vi "Init State.vi"(5 "Queue in":refnum<queue>, 9 "Test Results in":T1, 11 "error in (no error)":errorcluster) -> (4 ".NET Refnum out":refnum<k24>, 10 "Test Results out":T1, 15 "error out":errorcluster)   [LabVIEW 2016]
doc: "This VI Initializes the GEA2 bus, and sets the reference to the GEA2 Functional Global Variable."
uses:
  C:/Automation/DLLs/PC Dot Net/GeaCommunication.dll
  controls/Test Results.ctl
  C:/Program Files (x86)/National Instruments/LabVIEW 2016/examples/Design Patterns/Queued Message Handler/support/QMH Fundamentals - Message Cluster.ctl
  <vilib>/Utility/error.llb/Error Cluster From Error Code.vi
  <vilib>/ErrorRing/Error Ring.xnode
  Common/LabVIEW GEA2 Toolkit/LabVIEW_GEA2_Toolkit.lvlibp
  Automation/Product Specific/Clothes Care/TL27/Projects/TL27.lvlib
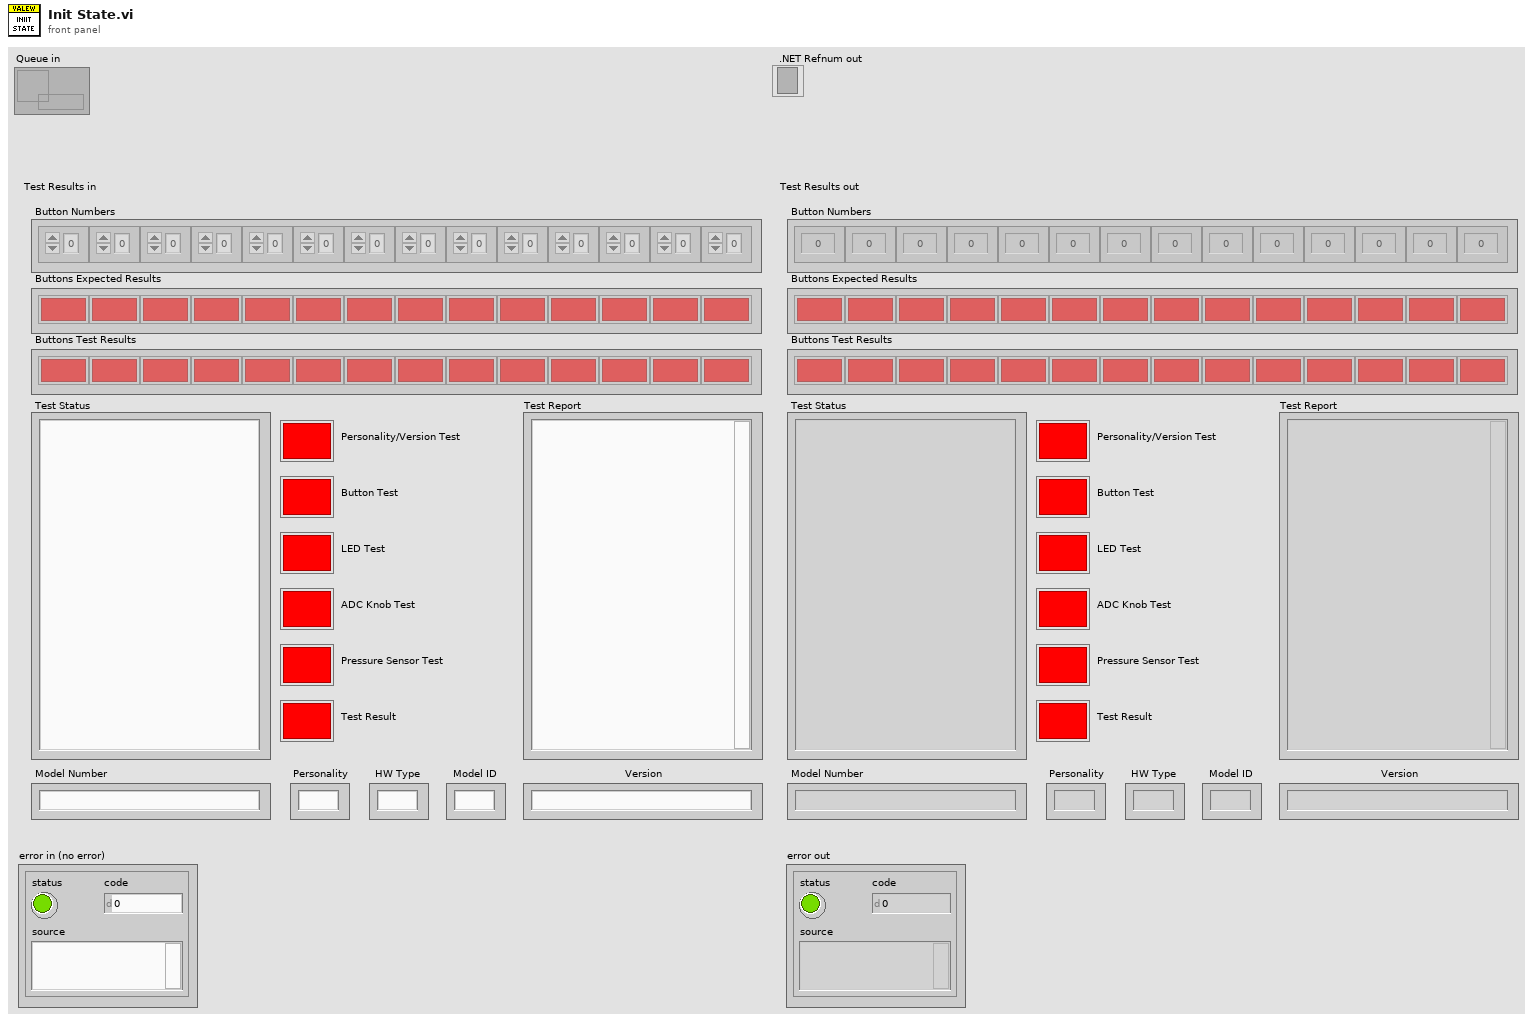
[diagram p1: front panel]
types:
  T1 = typedef "Test Results.ctl" = cluster{"Test Status":string, "Personality/Version Test ":bool, "Test Report":string, "Model Number":string, "Button Numbers":i32[], "Buttons Test Results":bool[], "Buttons Expected Results":bool[], "Model ID":string, "Personality":string, "HW Type":string, "Version":string, "Button Test":bool, "LED Test":bool, "ADC Knob Test":bool, "Pressure Sensor Test":bool, "Test Result":bool}
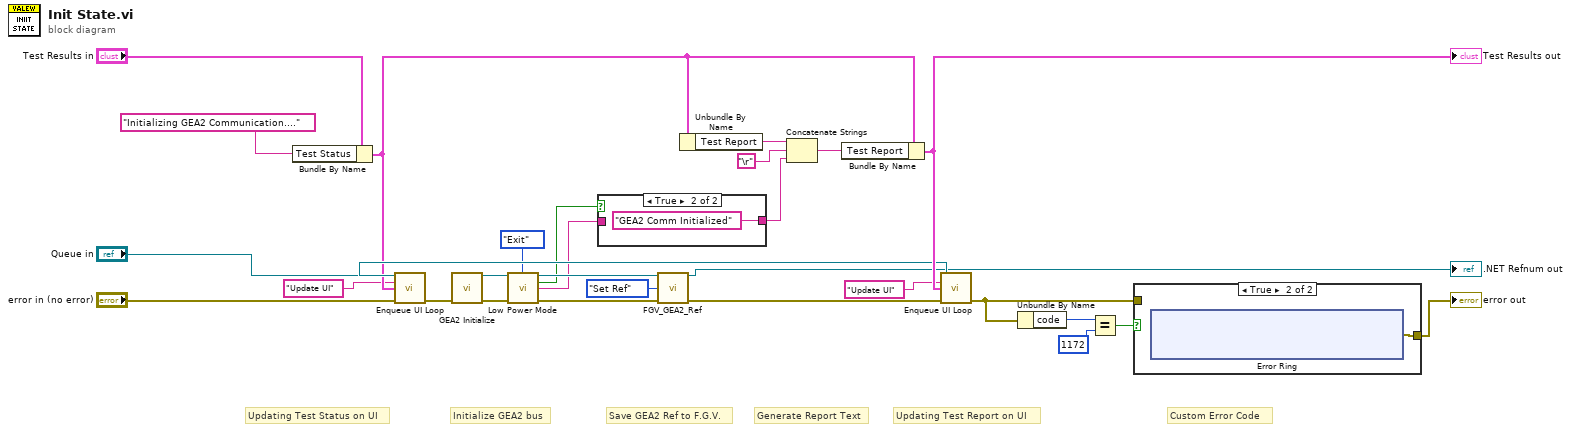
[diagram p0: block diagram]
diagram:
  # "Custom Error Code"
  # "Generate Report Text"
  # "Updating Test Status on UI"
  # "Updating Test Report on UI"
  # "Save GEA2 Ref to F.G.V."
  # "Initialize GEA2 bus"
  n1 = Bundle By Name(cluster="Test Results in", "Test Status"="Initializing GEA2 Communication....") -> (w22:T1)
  n2 = call "Enqueue UI Loop.vi"("UI Que In"="Queue in", "Message"="Update UI", "Test Results"=w22, "error in (no error)"="error in (no error)") -> ("UI Queue Out"=w24:refnum<queue>, "error out"=w20:errorcluster)  [unwired: 10 in]
  n3 = call "GEA2 Initialize.vi"("error in"=w20) -> ("GEA2 Reference Out"=w15:refnum<k24>, "error out"=w16:errorcluster)  [unwired: 12 in, 1 out]
  n4 = call "Low Power Mode.vi"("GEA2 Reference In"=w15, "Action"=enum16{"Enter", "Exit"}."Exit", "Error In"=w16) -> ("GEA2 Reference Out"=w28:refnum<k24>, "Pass/Fail?"=w18:bool, "Report Text"=w19:string, "Error Out"=w23:errorcluster)  [unwired: 9 in]
  n5 = case shown="True" w18 {
    tunnel: [w30 "GEA2 Comm Initialized"] -> w21
    tunnel: w19 -> [w30 _]
    frame False {
    }
    frame True {
    }
  }
  n6 = call "FGV_GEA2_Ref.vi"("GEA2 Reference In"=w28, "Action"=enum16{"Set Ref", "Get Ref"}."Set Ref", "Error In"=w23) -> ("GEA2 Reference Out"=→".NET Refnum out":refnum<k24>, "Error Out"=w27:errorcluster)  [unwired: 11 in]
  n7 = Unbundle By Name(w22) -> ("Test Report"=w9:string)
  n8 = Concatenate Strings(w9, "\r", w21) -> (w7:string)
  n9 = Bundle By Name(cluster=w22, "Test Report"=w7) -> (w26:T1)
  "Test Results out" <- w26
  n10 = call "Enqueue UI Loop.vi"("UI Que In"=w24, "Message"="Update UI", "Test Results"=w26, "error in (no error)"=w27) -> ("error out"=w2:errorcluster)  [unwired: 10 in, 1 out]
  n11 = Unbundle By Name(w2) -> ("code"=w6:i32)
  n12 = Equal?(x=w6, y=1172) -> (x = y?=w4:bool)
  n13 = case shown="True" w4 {
    tunnel: [w32 w33] -> w1
    tunnel: w2 -> [w32 _]
    frame False {
    }
    frame True {
      n14 = xnode "Error Ring"() -> ("error out"=w33:errorcluster)
    }
  }
  "error out" <- w1
